vi "Read Text from Text File.vi"(0 "Text and direction IN":T1, 7 "Text IN":string, 9 "Path":path, 11 "error in (no error)":errorcluster) -> (4 "Text and direction OUT":T1, 8 "Text OUT":string, 15 "error out":errorcluster)   [LabVIEW 2019, in "Exaprom PDF.lvlib"]
doc: "ASCII or UNICODE Text File\n\nDeveloped by Jean-Marc Simard\nCopyright © 2012, Exaprom Inc.\nAll rights reserved.\nLicense: BSD\n\nWith iTextSharp 4.1.6 (http://itextsharp.sourceforge.net)\nunder Mozilla Public License Version 1.1\n(http://www.mozilla.org/MPL/MPL-1.1.html)"
uses:
  Controls/Text Controls/Unicode/Type and run direction.ctl
  Exaprom PDF.lvlib
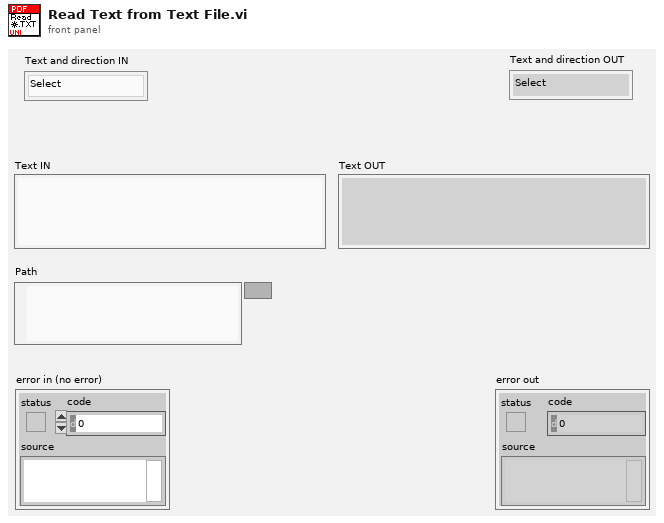
[diagram p1: front panel]
types:
  T1 = typedef "Exaprom PDF.lvlib/Type and run direction.ctl" = enum16{"Select", "ASCII", "UTF-16", "UTF-16 (default)", "UTF-16 (LTR)", "UTF-16 (RTL)"}
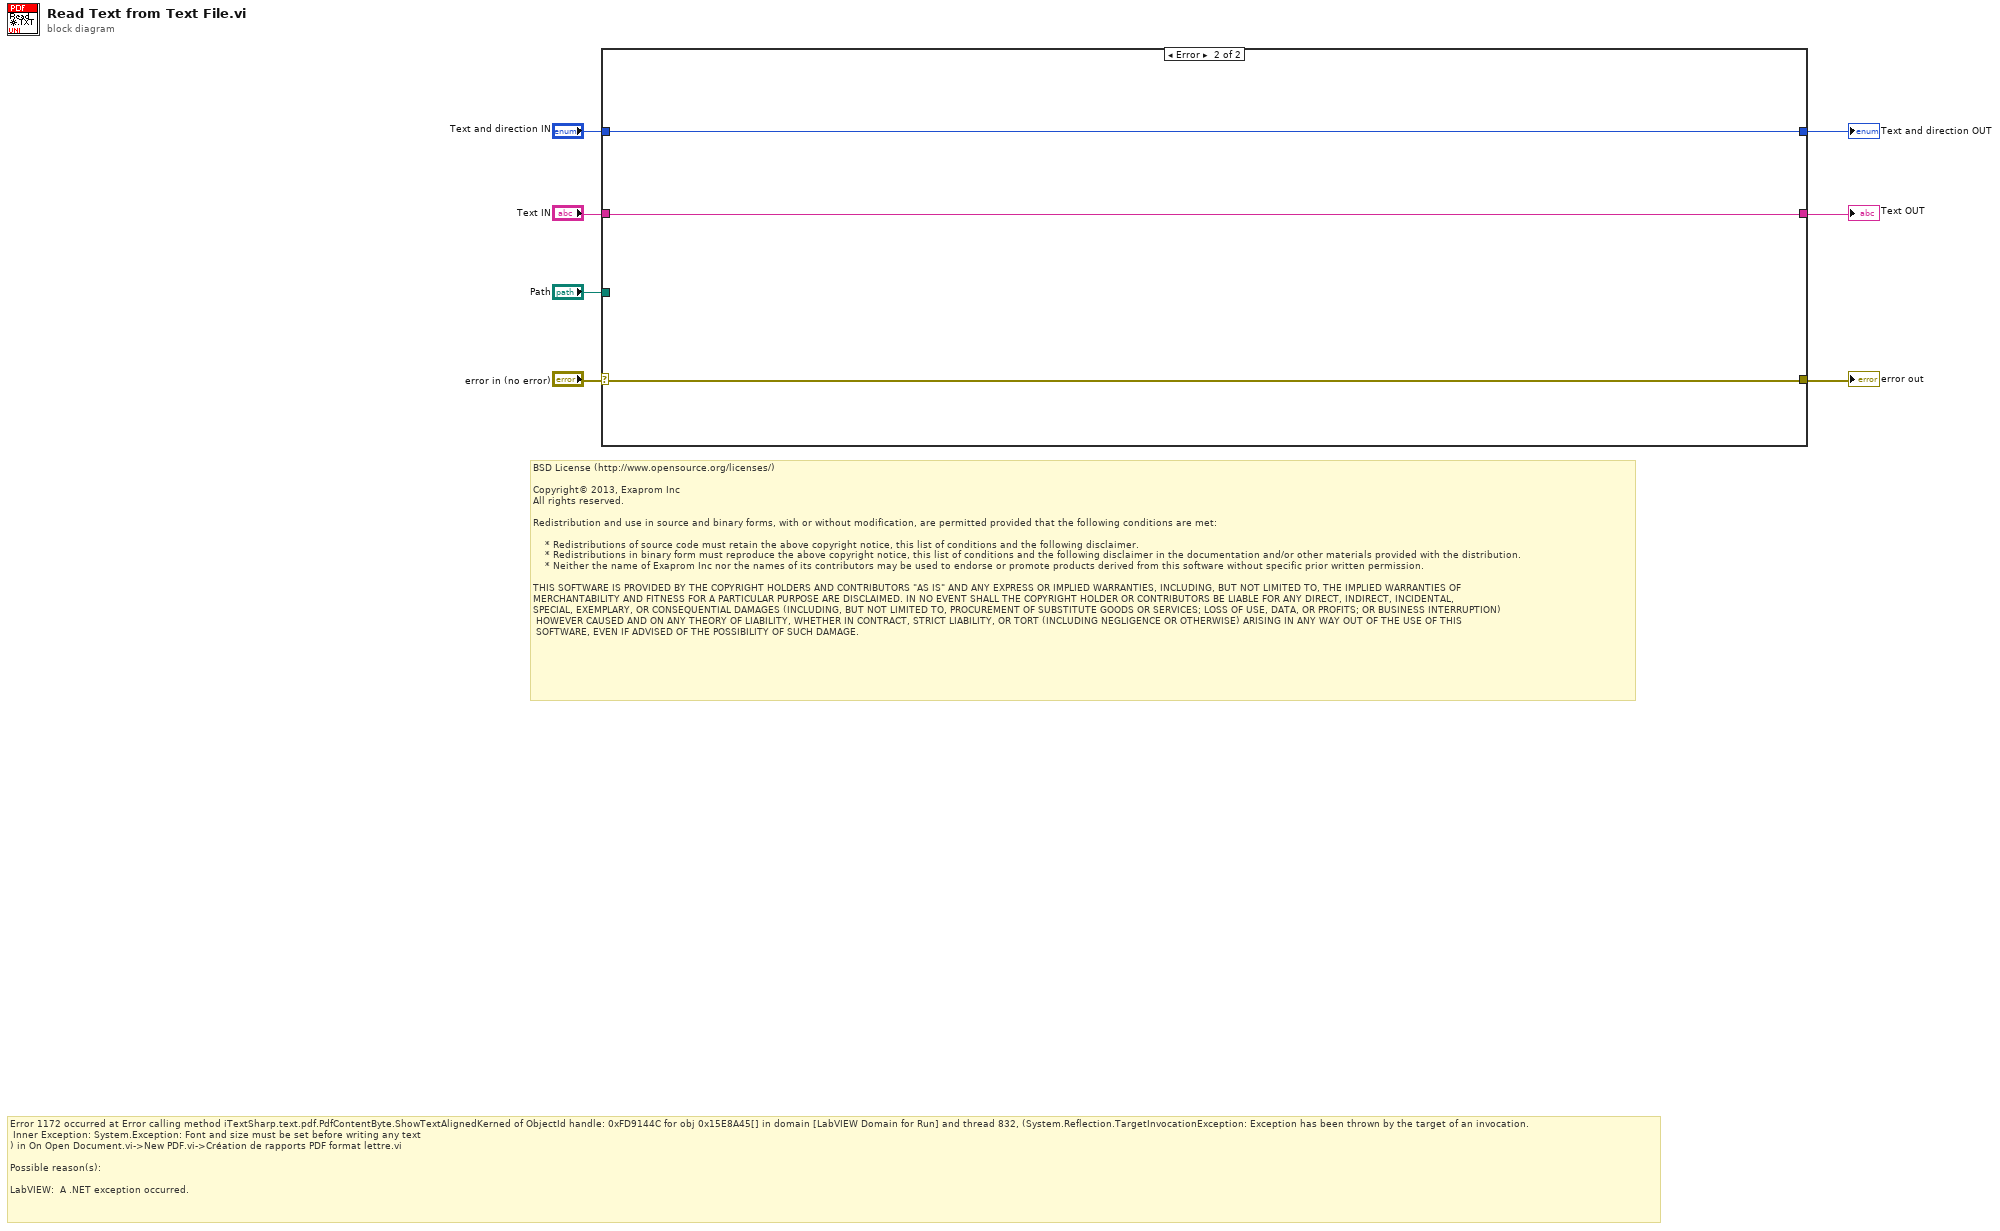
[diagram p0: block diagram]
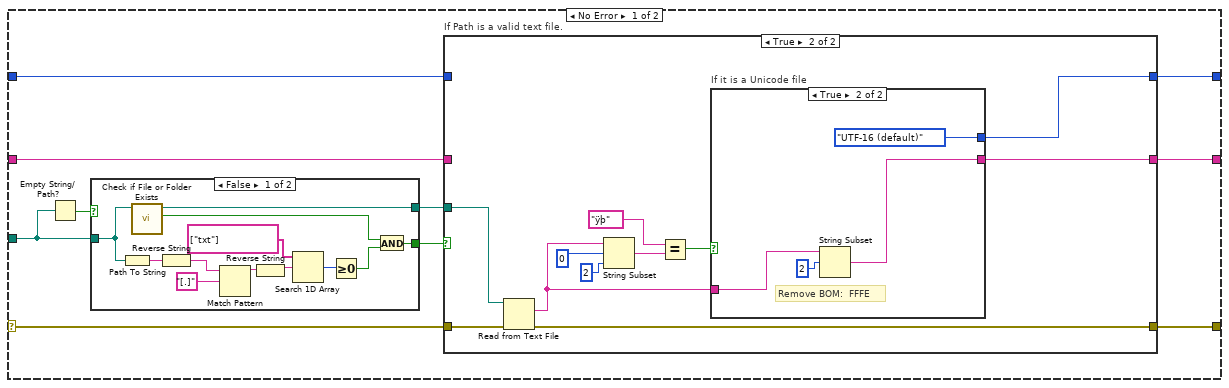
[diagram p2: hidden frame]
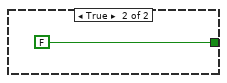
[diagram p3: hidden frame]
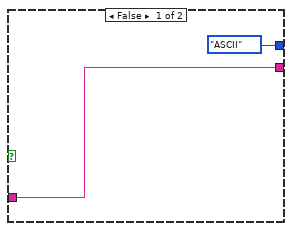
[diagram p5: hidden frame]
diagram:
  # "Error 1172 occurred at Error calling method iTextSharp.text.pdf.PdfContentByte.ShowTextAlignedKerned of ObjectId handle: 0xFD9144C for obj 0x15E8A45[] in domain [LabVIEW Domain for Run] and thread 832, (System.Reflection.TargetInvocationException: Exception has been thrown by the target of an invocation.\n\tInner Exception: System.Exception: Font and size must be set before writing any text\n) in On Open Document.vi->New PDF.vi->Création de rapports PDF format lettre.vi\n\nPossible reason(s):\n\nLabVIEW:  A .NET exception occurred."
  # "BSD License (http://www.opensource.org/licenses/)\n\nCopyright© 2013, Exaprom Inc\nAll rights reserved.\n\nRedistribution and use in source and binary forms, with or without modification, are permitted provided that the following conditions are met:\n\n    * Redistributions of source code must retain the above copyright notice, this list of conditions and the following disclaimer.\n    * Redistributions in binary form must reproduce the above copyright notice, this list of conditions and the following disclaimer in the documentation and/or other materials provided with the distribution.\n    * Neither the name of Exaprom Inc nor the names of its contributors may be used to endorse or promote products derived from this software without specific prior written permission.\n\nTHIS SOFTWARE IS PROVIDED BY THE COPYRIGHT HOLDERS AND CONTRIBUTORS \"AS IS\" AND ANY EXPRESS OR IMPLIED WARRANTIES, INCLUDING, BUT NOT LIMITED TO, THE IMPLIED WARRANTIES OF \nMERCHANTABILITY AND FITNESS FOR A PARTICULAR PURPOSE ARE DISCLAIMED. IN NO EVENT SHALL THE COPYRIGHT HOLDER OR CONTRIBUTORS BE LIABLE FOR ANY DIRECT, INDIRECT, INCIDENTAL,\nSPECIAL, EXEMPLARY, OR CONSEQUENTIAL DAMAGES (INCLUDING, BUT NOT LIMITED TO, PROCUREMENT OF SUBSTITUTE GOODS OR SERVICES; LOSS OF USE, DATA, OR PROFITS; OR BUSINESS INTERRUPTION)\n HOWEVER CAUSED AND ON ANY THEORY OF LIABILITY, WHETHER IN CONTRACT, STRICT LIABILITY, OR TORT (INCLUDING NEGLIGENCE OR OTHERWISE) ARISING IN ANY WAY OUT OF THE USE OF THIS\n SOFTWARE, EVEN IF ADVISED OF THE POSSIBILITY OF SUCH DAMAGE."
  n1 = case shown="Error" "error in (no error)" {
    selector: "error in (no error)" -> [w17 w53]
    tunnel: [w16 w53] -> w7
    tunnel: "Path" -> [w8 _]
    tunnel: "Text and direction IN" -> [w15 w52]
    tunnel: [w14 w52] -> w3
    tunnel: [w13 w51] -> w2
    tunnel: "Text IN" -> [w12 w51]
    frame No Error {
      n2 = Empty String/Path?(string/path=w8) -> (empty?=w9:bool)
      n3 = case shown="False" w9 {
        tunnel: w8 -> [w20 _]
        tunnel: [w19 FALSE] -> w11
        tunnel: [w18 _] -> w10
        frame False {
          n4 = Path To String(path=w20) -> (string=w26:string)
          n5 = call <vilib>:"Check if File or Folder Exists.vi"("path"=w20) -> ("file or folder exists?"=w27:bool, "dup path"=w18:path)  [unwired: 1 in, 8 out]
          n6 = Reverse String(1:w26) -> (0:w24:string)
          n7 = Match Pattern(string=w24, regular expression="[.]") -> (before substring=w22:string)  [unwired: 4 out]
          n8 = Reverse String(1:w22) -> (0:w21:string)
          n9 = Search 1D Array(1D array=string[] ["txt"], element=w21) -> (index of element=w28:i32)  [unwired: 1 out]
          n10 = Greater Or Equal To 0?(x=w28) -> (x >= 0?=w29:bool)
          n11 = And(x=w27, y=w29) -> (x .and. y?=w19:bool)
        }
        frame True {
        }
      }
      n12 = case "If Path is a valid text file." shown="True" w11 {
        tunnel: w17 -> [w31 w44]
        tunnel: [w31 w43] -> w16
        tunnel: w15 -> [w32 _]
        tunnel: [w32 w34] -> w14
        tunnel: [w33 w36] -> w13
        tunnel: w12 -> [w33 _]
        tunnel: w10 -> [_ w35]
        frame False {
        }
        frame True {
          n13 = Read from Text File(file (use dialog)=w35, error in=w44) -> (text=w37:string, error out=w43:errorcluster)  [unwired: 2 in, 2 out]
          n14 = String Subset(string=w37, offset (0)=0, length (rest)=2 ("length (rest)")) -> (substring=w40:string)
          n15 = Equal?(x="ÿþ", y=w40) -> (x = y?=w38:bool)
          n16 = case "If it is a Unicode file" shown="True" w38 {
            tunnel: w37 -> [w46 w49]
            tunnel: [w46 w48] -> w36
            tunnel: [Type_and_run_direction."ASCII" ("Text and direction OUT") Type_and_run_direction."UTF-16 (default)" ("Text and direction OUT")] -> w34
            frame False {
            }
            frame True {
              # "Remove BOM:  FFFE"
              n17 = String Subset(string=w49, offset (0)=2) -> (substring=w48:string)  [unwired: 1 in]
            }
          }
        }
      }
    }
    frame Error {
    }
  }
  "error out" <- w7
  "Text and direction OUT" <- w3
  "Text OUT" <- w2
